vi "OpenTestImage.vi"() -> ()   [LabVIEW 2011]
uses:
  Debug/cudaqi-labview.dll
panel:
  in  "OK Button":bool
  out "Numeric Indicator 2":dbl
  out "Numeric Indicator":dbl
  out "String":string
  out "Original":T1(plugin-control)
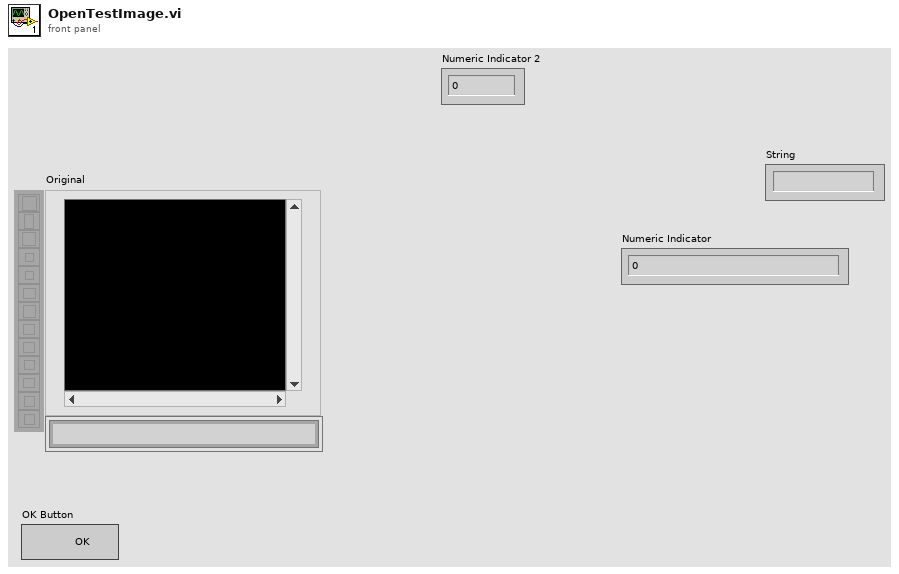
[diagram p1: front panel]
types:
  T1 = typedef "IMAQ Image.ctl" = refnum<image>
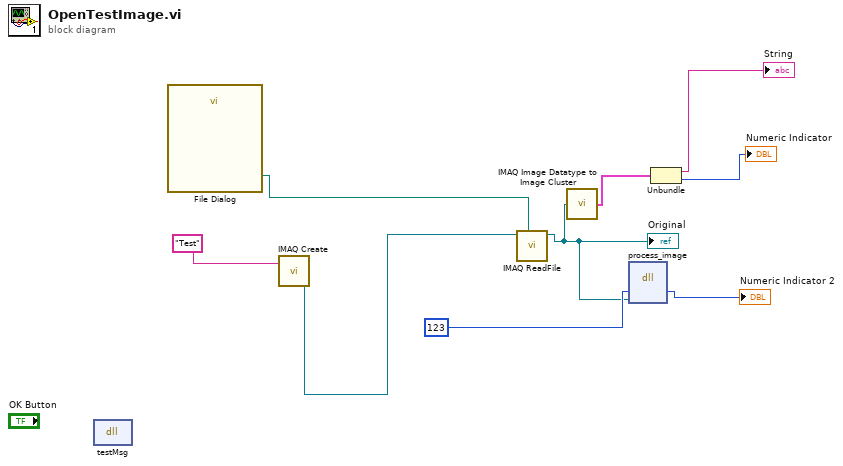
[diagram p0: block diagram]
diagram:
  n1 = dll-call lib="D:/jpcnossen/cudaqi-tracker/Debug/cudaqi-labview.dll" fn="testMsg"() -> ()  [unwired: 4 in, 2 out]
  n2 = call "File Dialog"() -> ("selected path"=w9:path)  [unwired: 12 in, 3 out]
  n3 = call "IMAQ Create"("Image Name"="Test" ("String")) -> ("New Image"=w7:T1)  [unwired: 4 in, 1 out]
  n4 = call "IMAQ ReadFile"("File Path"=w9, "Image"=w7) -> ("Image Out"=w5:T1)  [unwired: 5 in, 4 out]
  "Original" <- w5
  n5 = call <vilib>:"IMAQ Image Datatype to Image Cluster.vi"("Image"=w5) -> ("Image (dup)"=w4:cluster{string, u32})
  n6 = dll-call lib="D:/jpcnossen/cudaqi-tracker/Debug/cudaqi-labview.dll" fn="process_image"("position"=123, "image"=w5) -> ("position"=→"Numeric Indicator 2":i32)  [unwired: 5 in, 2 out]
  n7 = Unbundle(w4) -> (→"String":string, →"Numeric Indicator":u32)
